vi "Debounce.vi"(1 "Reset":bool, 2 "Input":bool, 3 "Num samples":i32=10) -> (0 "Output":bool)   [LabVIEW 2016, in "ArgosLib.lvlib"]
uses:
  ArgosLib.lvlib
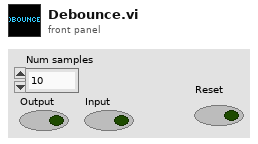
[diagram p1: front panel]
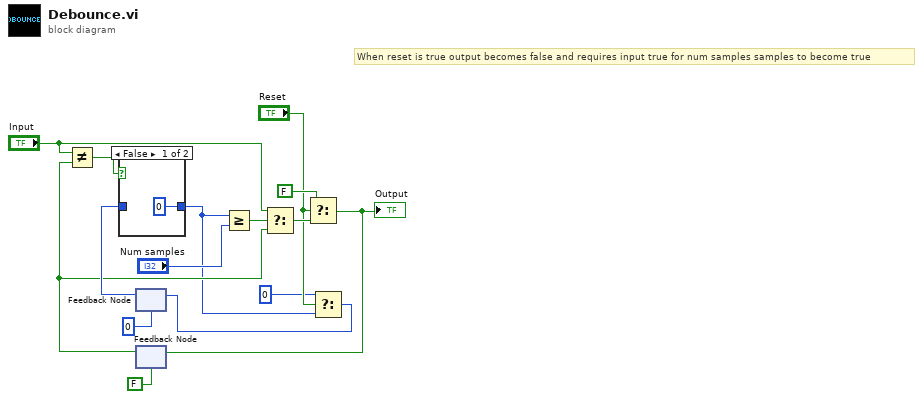
[diagram p0: block diagram]
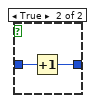
[diagram p2: hidden frame]
diagram:
  # "When reset is true output becomes false and requires input true for num samples samples to become true"
  n1 = feedback #1(0) -> (w11:i32)
  n2 = feedback #2(FALSE ("Input")) -> (w9:bool)
  n3 = Not Equal?(x="Input", y=w9) -> (x != y?=w15:bool)
  n4 = case shown="False" w15 {
    tunnel: w11 -> [_ w18]
    tunnel: [0 w17] -> w4
    frame False {
    }
    frame True {
      n5 = Increment(x=w18) -> (x+1=w17:i32)
    }
  }
  n6 = Greater Or Equal?(x=w4, y="Num samples") -> (x >= y?=w13:bool)
  n7 = Select(t="Input", s=w13, f=w9) -> (s? t:f=w6:bool)
  n8 = Select(t=FALSE, s="Reset", f=w6) -> (s? t:f=w7:bool)
  "Output" <- w7
  n9 = feedback-in #2(w7) -> ()
  n10 = Select(t=0, s="Reset", f=w4) -> (s? t:f=w1:i32)
  n11 = feedback-in #1(w1) -> ()
